vi "Integrator w Limits.vi"(4 "Initial Condition":sgl, 5 "lower limit":sgl, 6 "Initialize (F)":bool, 7 "upper limit":sgl, 8 "dt [s]":sgl, 11 "x":sgl) -> (3 "Result":sgl)   [LabVIEW 2016, in "NI-PCG Vehicle Model.lvlib"]
uses:
  NI-PCG Vehicle Model.lvlib
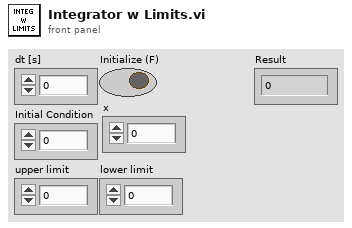
[diagram p1: front panel]
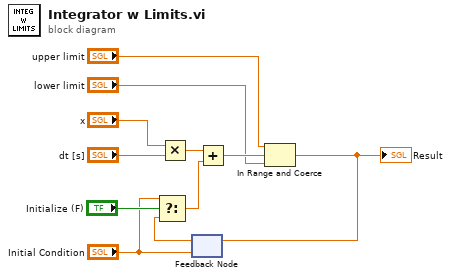
[diagram p0: block diagram]
diagram:
  n1 = Multiply(x="x", y="dt [s]") -> (x*y=w11:sgl)
  n2 = feedback #1("Initial Condition") -> (w7:sgl)
  n3 = Select(t="Initial Condition", s="Initialize (F)", f=w7) -> (s? t:f=w9:sgl)
  n4 = Add(x=w11, y=w9) -> (x+y=w3:sgl)
  n5 = In Range and Coerce(upper limit="upper limit", x=w3, lower limit="lower limit") -> (coerced(x)=w4:sgl)  [unwired: 1 out]
  "Result" <- w4
  n6 = feedback-in #1(w4) -> ()
